vi "String - Check Empty Cells.vi"(10 "Exclude Last Row (T)":bool=TRUE, 11 "ItemNames":string[][](array[string])) -> (1 "Rows > 0":bool, 2 "Location of Empty Cell (R,C)":i32[][](array[numeric]), 3 "Empty Cell(s)":bool)   [LabVIEW 2013]
panel:
  out "sum":i32
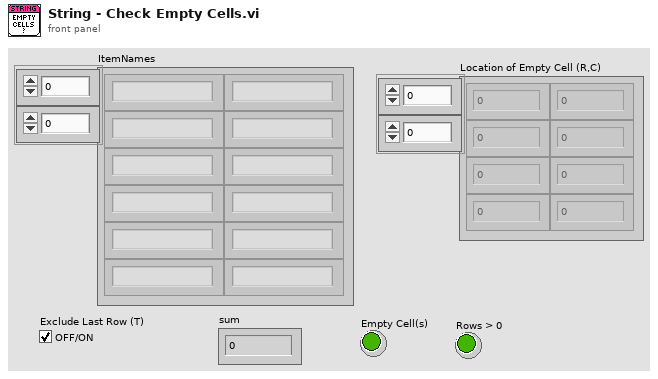
[diagram p1: front panel]
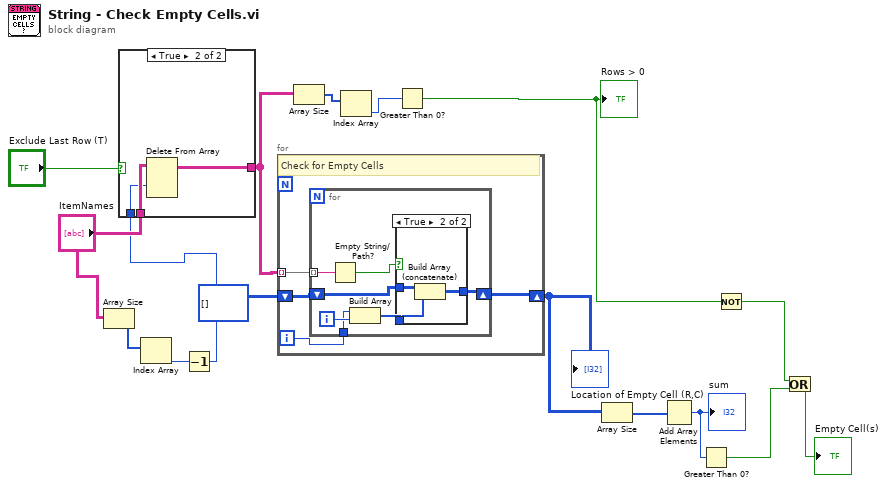
[diagram p0: block diagram]
diagram:
  n1 = Array Size(array="ItemNames") -> (size(s)=w15:i32[])
  n2 = Index Array(array=w15) -> (element=w14:i32)  [unwired: 1 in]
  n3 = Decrement(x=w14) -> (x-1=w9:i32)
  n4 = case shown="True" "Exclude Last Row (T)" {
    tunnel: "ItemNames" -> [w17 w20]
    tunnel: w9 -> [_ w18]
    tunnel: [w17 w19] -> w7
    frame False {
    }
    frame True {
      n5 = Delete From Array(array=w20, index (row)=w18) -> (array with subset deleted=w19:string[][])  [unwired: 2 in, 1 out]
    }
  }
  n6 = for {
    tunnel: w7 -> [w24] mode=indexing
    shift-right: [w22] -> w13
    shift-left: i32[][] [] -> [w23]
    i -> [w21]
    # "Check for Empty Cells"
    n7 = for {
      tunnel: w24 -> [w31] mode=indexing
      shift-right: [w27] -> w22
      shift-left: w23 -> [w30]
      tunnel: w21 -> [w26]
      i -> [w29]
      n8 = Empty String/Path?(string/path=w31) -> (empty?=w25:bool)
      n9 = Build Array(w26, w29) -> (w28:i32[])
      n10 = case shown="True" w25 {
        tunnel: w30 -> [w32 w35]
        tunnel: w28 -> [_ w34]
        tunnel: [w32 w33] -> w27
        frame False {
        }
        frame True {
          n11 = Build Array (concatenate)(w35, w34) -> (w33:i32[][])
        }
      }
    }
  }
  "Location of Empty Cell (R,C)" <- w13
  n12 = Array Size(array=w7) -> (size(s)=w6:i32[])
  n13 = Index Array(array=w6) -> (element=w5:i32)  [unwired: 1 in]
  n14 = Greater Than 0?(x=w5) -> (x > 0?=w4:bool)
  "Rows > 0" <- w4
  n15 = Array Size(array=w13) -> (size(s)=w12:i32[])
  n16 = Add Array Elements(numeric array=w12) -> (sum=w11:i32)
  "sum" <- w11
  n17 = Greater Than 0?(x=w11) -> (x > 0?=w2:bool)
  n18 = Not(x=w4) -> (.not. x?=w3:bool)
  n19 = Or(x=w3, y=w2) -> (x .or. y?=→"Empty Cell(s)":bool)
